vi "Request Worker Show.vi"(8 "error in (no error)":errorcluster, 10 "index":i32, 11 "Comm Interface in":refnum<class "Comm Interface.lvclass">) -> (0 "error out":errorcluster, 3 "Comm Interface out":refnum<class "Comm Interface.lvclass">)   [LabVIEW 2017, in "Comm Interface.lvlib" / "Comm Interface.lvclass"]
uses:
  Comm Interface.lvclass
  Message Interface/Command/Command.lvclass
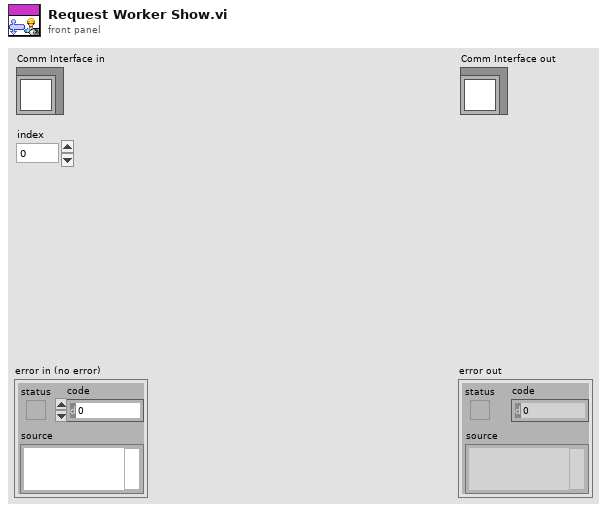
[diagram p1: front panel]
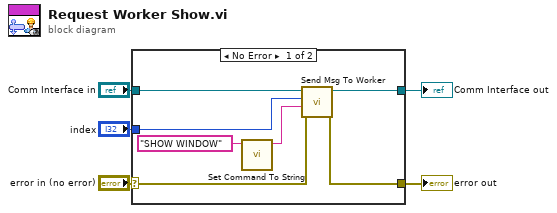
[diagram p0: block diagram]
diagram:
  n1 = case shown="No Error" "error in (no error)" {
    selector: "error in (no error)" -> [w7 w14]
    tunnel: [w6 w14] -> w4
    tunnel: [w10 w13] -> w2
    tunnel: "Comm Interface in" -> [w11 w13]
    tunnel: "index" -> [w8 _]
    frame No Error {
      n2 = call "Set Command To String.vi"("Command"="SHOW WINDOW") -> ("data string"=w9:string)  [unwired: 10 in]
      n3 = call "Send Msg To Worker.vi"("error in (no error)"=w7, "Message"=w9, "index"=w8, "Comm Interface in"=w11) -> ("error out"=w6:errorcluster, "Comm Interface out"=w10:refnum<class "Comm Interface.lvclass">)  [unwired: 6 in]
    }
    frame Error {
    }
  }
  "error out" <- w4
  "Comm Interface out" <- w2
